vi "羽状图.vi"() -> ()   [LabVIEW 2012]
uses:
  <vilib>/Math Plots/2D Math Plots/2D Feather/2D Feather XCtrl/2D Feather.xctl
  <vilib>/Math Plots/2D Math Plots/2D Feather/2D Feather Datatype/Public/Plot Helper (Vector).vi
  <vilib>/imath/engines/lvmath2/RunTimeEngine/ErrorHandling/NIMS_Finalize Error.vi
  <vilib>/imath/engines/lvmath2/RunTimeEngine/Managers/WorkSpace/UID Generator.vi
  <vilib>/imath/engines/lvmath2/RunTimeEngine/Managers/SymbolTable/Clear UID.vi
  <vilib>/imath/engines/lvmath2/RunTimeEngine/NodeEndStatement/NIMS_NodeEndStatement_Output.vi
  <instcachedir>/0/NIMS_NodeEndStatement_Output_53EC0D466D134D7ABD903AC30B43404B.lvgen/NIMS_NodeEndStatement_Output_53EC0D466D134D7ABD903AC30B43404B_005.vi
  <vilib>/imath/engines/lvmath2/RunTimeEngine/RangeToken/NIMS_Range.vi
  <instcachedir>/0/NIMS_Range_3104F3C74E39439AB2C0407E7DA2F64D.lvgen/NIMS_Range_3104F3C74E39439AB2C0407E7DA2F64D_001.vi
  <vilib>/imathl/engines/lvmath/Functions/Error Handling/Create Error.vi
  <vilib>/imath/engines/lvmath2/RunTimeEngine/ArithmeticOperatorToken/NIMS_ArithmeticOperator_times.vi
  <instcachedir>/0/NIMS_ArithmeticOperator_times_1C9874CB0A2E40D3A609F62CD8BBF4DC.lvgen/NIMS_ArithmeticOperator_times_1C9874CB0A2E40D3A609F62CD8BBF4DC_000.vi
  <vilib>/imath/engines/lvmath2/RunTimeEngine/ArithmeticOperatorToken/NIMS_ArithmeticOperator_plus.vi
  <instcachedir>/0/NIMS_ArithmeticOperator_plus_8BD56D3B58F64DB5ABEB7224541A3CE7.lvgen/NIMS_ArithmeticOperator_plus_8BD56D3B58F64DB5ABEB7224541A3CE7_004.vi
  <vilib>/imath/engines/lvmath2/RunTimeEngine/ErrorHandling/NIMS_Create Error From Enums.vi
  <vilib>/imath/engines/lvmath2/RunTimeEngine/ArithmeticOperatorToken/NIMS_ArithmeticOperator_minus.vi
  <instcachedir>/0/NIMS_ArithmeticOperator_minus_E353D3D62E0E432C853B0E64BA14CDF8.lvgen/NIMS_ArithmeticOperator_minus_E353D3D62E0E432C853B0E64BA14CDF8_003.vi
  <vilib>/imath/engines/lvmath2/RunTimeEngine/BuiltInFunctions/feather/NIMS_feather(RV,RV).vi
  <vilib>/Math Plots/2D Math Plots/2D Feather/2D Feather Datatype/2D Feather Datatype.lvclass
  <vilib>/imath/engines/lvmath2/RunTimeEngine/Managers/SymbolTable/NIMS_WorkSpace.lvlib
panel:
  out "2D Feather":refnum<class "2D Plot Datatype.lvclass">[](xcontrol) caption="二维羽状图"
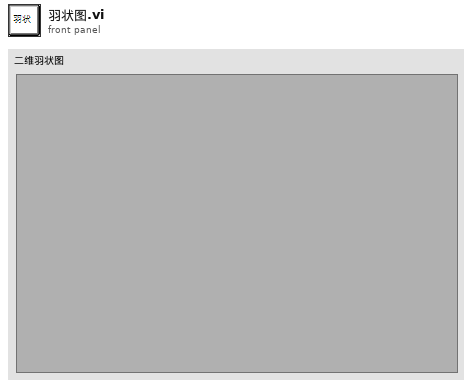
[diagram p1: front panel]
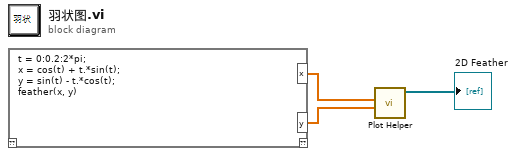
[diagram p0: block diagram]
diagram:
  n1 = mathscript code="t = 0:0.2:2*pi;\nx = cos(t) + t.*sin(t);\ny = sin(t) - t.*cos(t);\nfeather(x, y)"() -> ("x"=w2:dbl[], "y"=w1:dbl[])  [unwired: 1 in, 1 out]
  n2 = call-poly <vilib>:"Plot Helper.vi"("y vector"=w1, "x vector"=w2) -> ("2D Plot Class Obj Array out"=→"2D Feather":refnum<class "2D Plot Datatype.lvclass">[])  [unwired: 2 in, 7 out]
